vi "drive forward.vi"(6 "time out":i32=15000, 8 "error in (no error)":errorcluster, 9 "forward":bool=TRUE, 10 "desired distance":dbl, 11 "RobotDriveDevRef in":T1) -> (0 "error out":errorcluster, 3 "RobotDriveDevRef out":T1)   [LabVIEW 2016]
uses:
  <vilib>/Rock Robotics/WPI/RobotDrive/WPI_RobotDriveDevRef.ctl
  <vilib>/Rock Robotics/WPI/MotorControl/WPI_MotorControlDeviceRef.ctl
  <vilib>/Rock Robotics/WPI/MotorControl/WPI_MotorControlType.ctl
  <vilib>/Rock Robotics/SystemInterfaces/DIO/FPGA_DIOPWMChannel.ctl
  <vilib>/Rock Robotics/WPI/PWM/WPI_PWMDeadband.ctl
  <vilib>/Rock Robotics/WPI/RobotDrive/WPI_RobotDriveArcadeDrive_Standard(NoSaturation).vi
  <vilib>/Rock Robotics/Network Tables/NT Write Number.vi
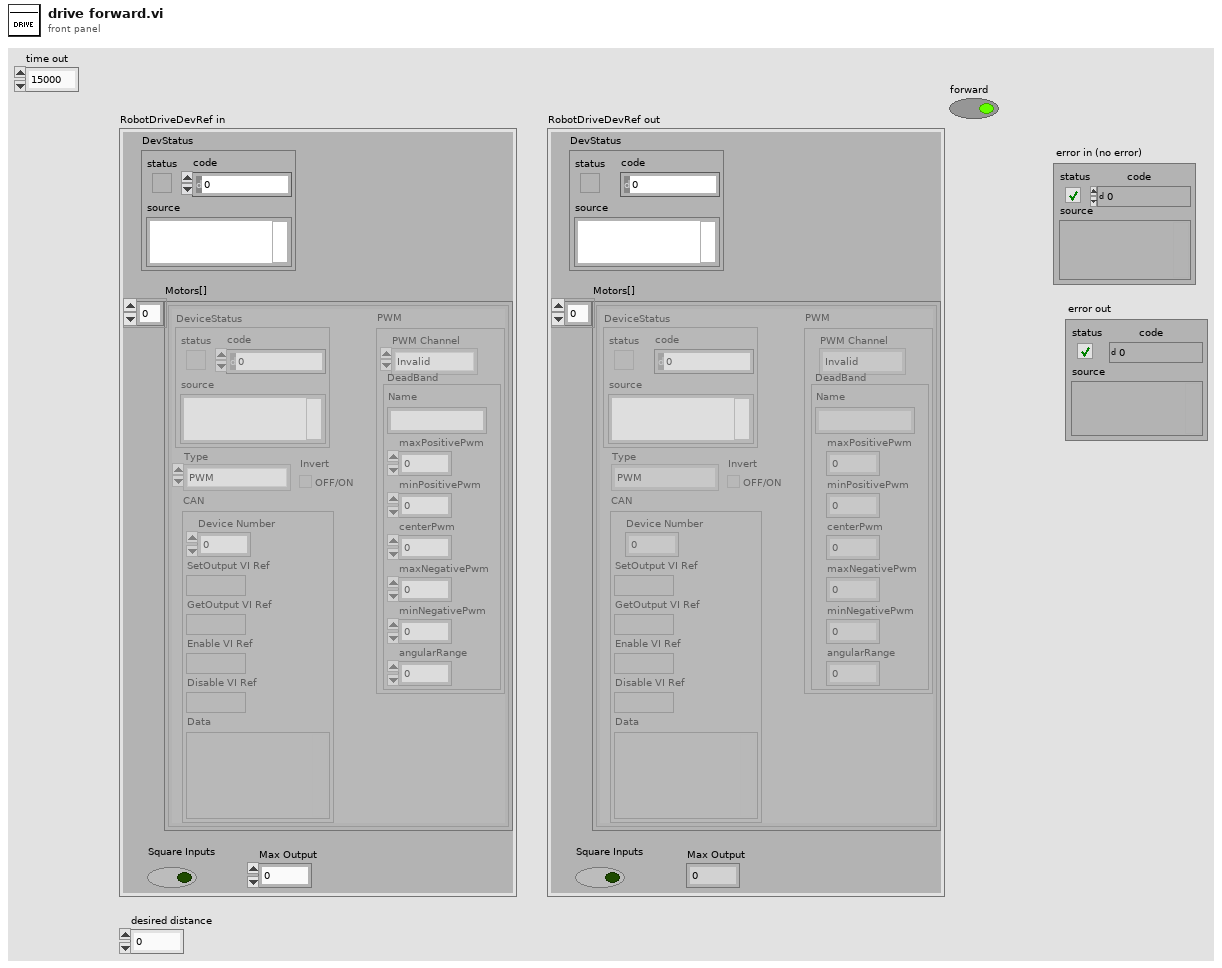
[diagram p1: front panel]
types:
  T1 = typedef "WPI_RobotDriveDevRef.ctl" = cluster{"DevStatus":errorcluster, "Motors[]":T2[], "Square Inputs":bool, "Max Output":dbl}
  T2 = typedef "WPI_MotorControlDeviceRef.ctl" = cluster{"DeviceStatus":errorcluster, "Type":T3, "PWM":cluster{"PWM Channel":T4, "DeadBand":T5}, "CAN":cluster{"Device Number":u8, "SetOutput VI Ref":variant, "GetOutput VI Ref":variant, "Enable VI Ref":variant, "Disable VI Ref":variant, "Data":variant}, "Invert":bool}
  T3 = typedef "WPI_MotorControlType.ctl" = enum16{"PWM", "CAN"}
  T4 = typedef "FPGA_DIOPWMChannel.ctl" = enum8{"PWM 0", "PWM 1", "PWM 2", "PWM 3", "PWM 4", "PWM 5", "PWM 6", "PWM 7", "PWM 8", "PWM 9", "PWM MXP 0", "PWM MXP 1", "PWM MXP 2", "PWM MXP 3", "PWM MXP 4", "PWM MXP 5", "PWM MXP 6", "PWM MXP 7", "PWM MXP 8", "PWM MXP 9", "Invalid"}
  T5 = typedef "WPI_PWMDeadband.ctl" = cluster{"Name":string, "maxPositivePwm":i32, "minPositivePwm":i32, "centerPwm":i32, "maxNegativePwm":i32, "minNegativePwm":i32, "angularRange":u16}
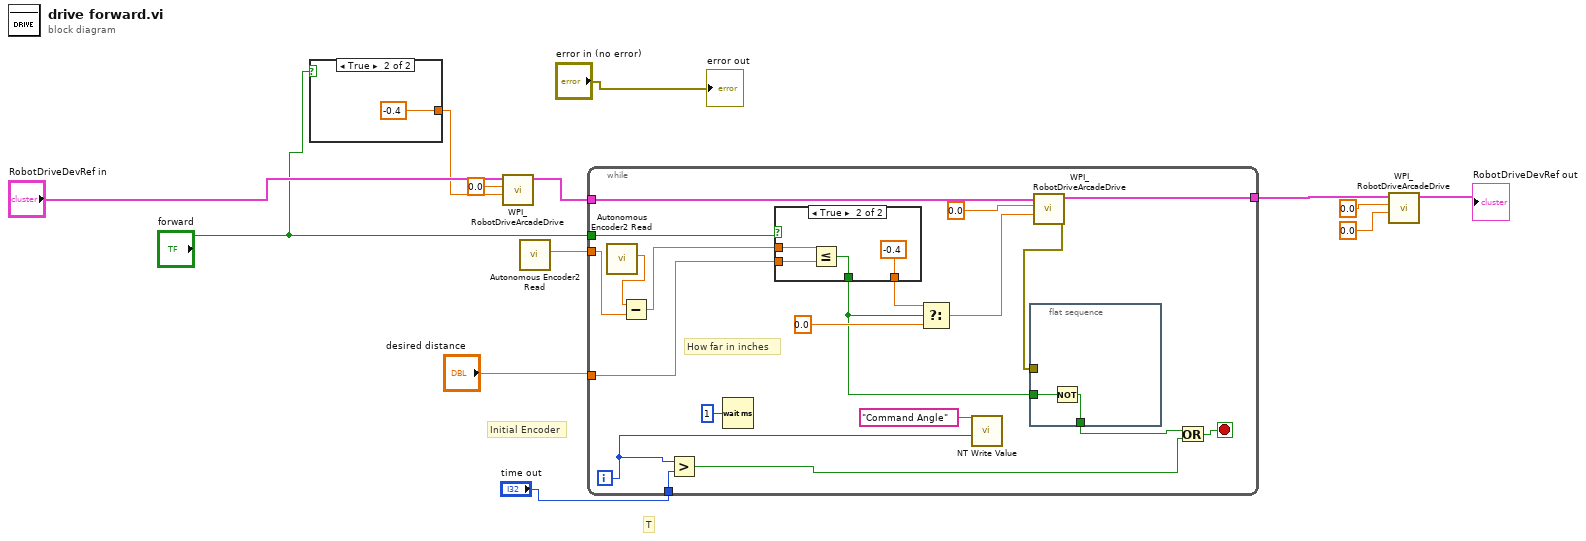
[diagram p0: block diagram]
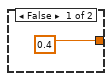
[diagram p2: hidden frame]
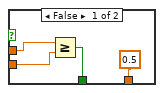
[diagram p3: hidden frame]
diagram:
  # "T"
  # "Initial Encoder"
  n1 = case shown="True" "forward" {
    tunnel: [0.4 ("t") -0.4 ("t")] -> w7
    frame False {
    }
    frame True {
    }
  }
  n2 = call-poly <vilib>:"WPI_RobotDriveArcadeDrive.vi"("Y axis value"=w7, "X axis value"=0.0, "RobotDriveDevRef"="RobotDriveDevRef in") -> ("RobotDriveDevRef"=w9:T1)  [unwired: 1 in, 7 out]
  n3 = call "Autonomous Encoder2 Read.vi"() -> ("Encoder Distance"=w11:dbl)  [unwired: 9 in, 2 out]
  n4 = while {
    tunnel: w9 -> [w31]
    tunnel: [w30] -> w3
    tunnel: "desired distance" -> [w28]
    tunnel: "forward" -> [w26]
    tunnel: w11 -> [w22]
    tunnel: "time out" -> [w16]
    i -> [w17]
    stop <- w18 stop-if-true
    # "How far in inches"
    n5 = call "Autonomous Encoder2 Read.vi"() -> ("Encoder Distance"=w23:dbl)  [unwired: 9 in, 2 out]
    n6 = Subtract(x=w23, y=w22) -> (x-y=w21:dbl)
    n7 = Greater?(x=w17, y=w16) -> (0:w19:bool)
    n8 = Wait (ms)(milliseconds to wait=u32 1) -> ()  [unwired: 1 out]
    n9 = case shown="True" w26 {
      tunnel: [0.5 ("t") -0.4 ("t")] -> w35
      tunnel: w21 -> [w37 w42]
      tunnel: w28 -> [w36 w41]
      tunnel: [w38 w40] -> w27
      frame False {
        n10 = Greater Or Equal?(x=w37, y=w36) -> (x >= y?=w38:bool)
      }
      frame True {
        n11 = Less Or Equal?(x=w42, y=w41) -> (x <= y?=w40:bool)
      }
    }
    n12 = Select(t=w35, s=w27, f=0.0) -> (s? t:f=w24:dbl)
    n13 = call-poly <vilib>:"NT Write Value.vi"("Numeric"=w17, "Name"="Command Angle") -> ()  [unwired: 9 in, 1 out]
    n14 = flat-sequence {
      tunnel: w27 -> [w45]
      tunnel: [w44] -> w20
      tunnel: w32 -> [_]
      frame #0 {
        n15 = Not(x=w45) -> (.not. x?=w44:bool)
      }
    }
    n16 = call-poly <vilib>:"WPI_RobotDriveArcadeDrive.vi"("Y axis value"=w24, "X axis value"=0.0, "RobotDriveDevRef"=w31) -> ("error out"=w32:errorcluster, "RobotDriveDevRef"=w30:T1)  [unwired: 6 in, 1 out]
    n17 = Or(x=w20, y=w19) -> (x .or. y?=w18:bool)
  }
  n18 = call-poly <vilib>:"WPI_RobotDriveArcadeDrive.vi"("Y axis value"=0.0, "X axis value"=0.0, "RobotDriveDevRef"=w3) -> ("RobotDriveDevRef"=→"RobotDriveDevRef out":T1)  [unwired: 1 in, 7 out]
  "error out" <- "error in (no error)"
